vi "GenericIMAQSetConfig.vi"(8 "Show error dialog (F)":bool=TRUE, 10 "Camera":T1={"Framerate (Hz)"=100, "Exposure time (us)"=100, "Image size"={"Width"=1280, "Height"=1024}, "Number of buffers"=30}, 11 "IMAQ Session In":refnum<k11>) -> (3 "IMAQ Session Out":refnum<k11>)   [LabVIEW 2011]
uses:
  Main/Camera/GenericCameraConfigType.ctl
  Global_GenericIMAQCamera_HardwareConfig.vi
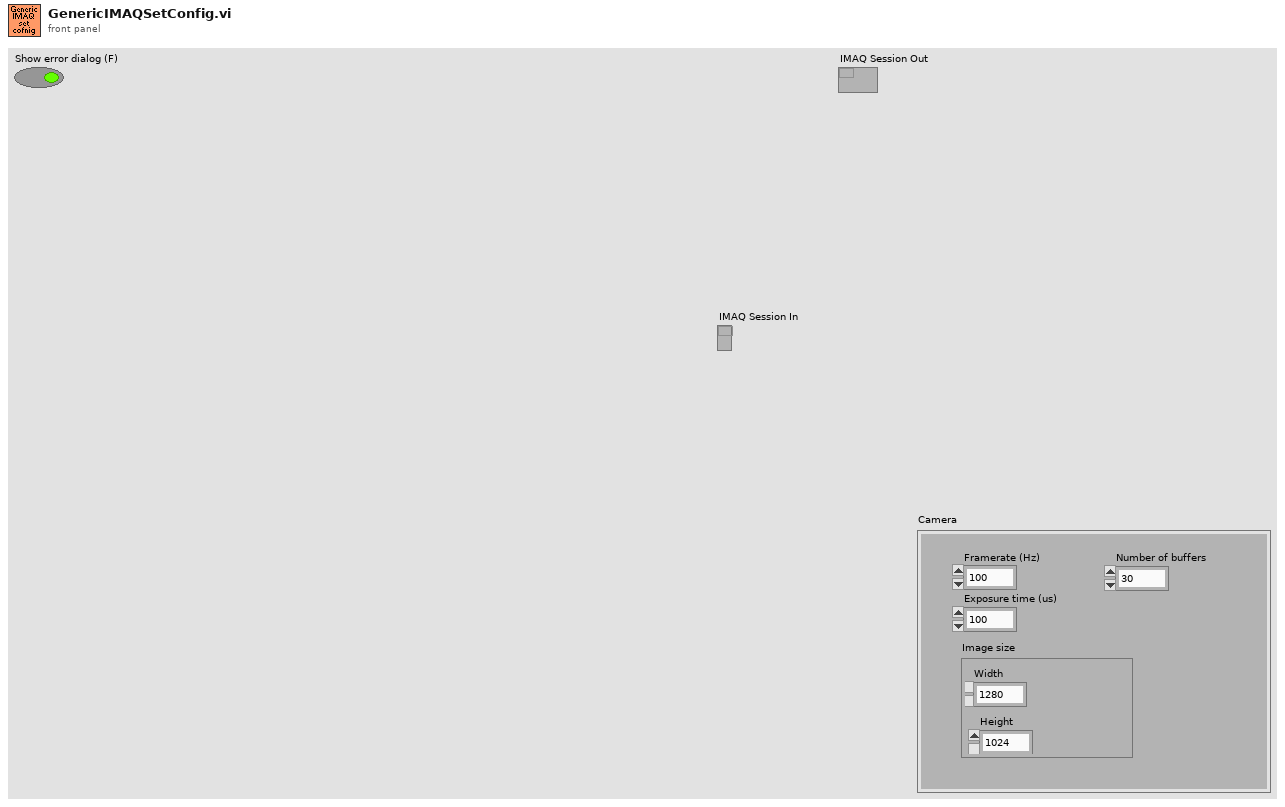
[diagram p1: front panel]
types:
  T1 = typedef "GenericCameraConfigType.ctl" = cluster{"Framerate (Hz)":i32, "Exposure time (us)":i32, "Image size":cluster{"Width":i32, "Height":i32}, "Number of buffers":i32}
  T2 = typedef "GenericIMAQHardwareConfig.ctl" = cluster{"Camera config mode":enum16{"Serial", "IMAQParam", "NoConfig"}, "Frame rate set cmd":string, "Exposure time set cmd":string, "Frame rate get cmd":string, "Exposure time get cmd":string, "IMAQ Identifier":string, "Serial return skip chars":i32, "Set width/height":string, "Set offset xy":string, "Get width":string, "Get height":string, "Get offset X":string, "Get offset Y":string, "Full frame size":cluster{"width":i32, "height":i32}}
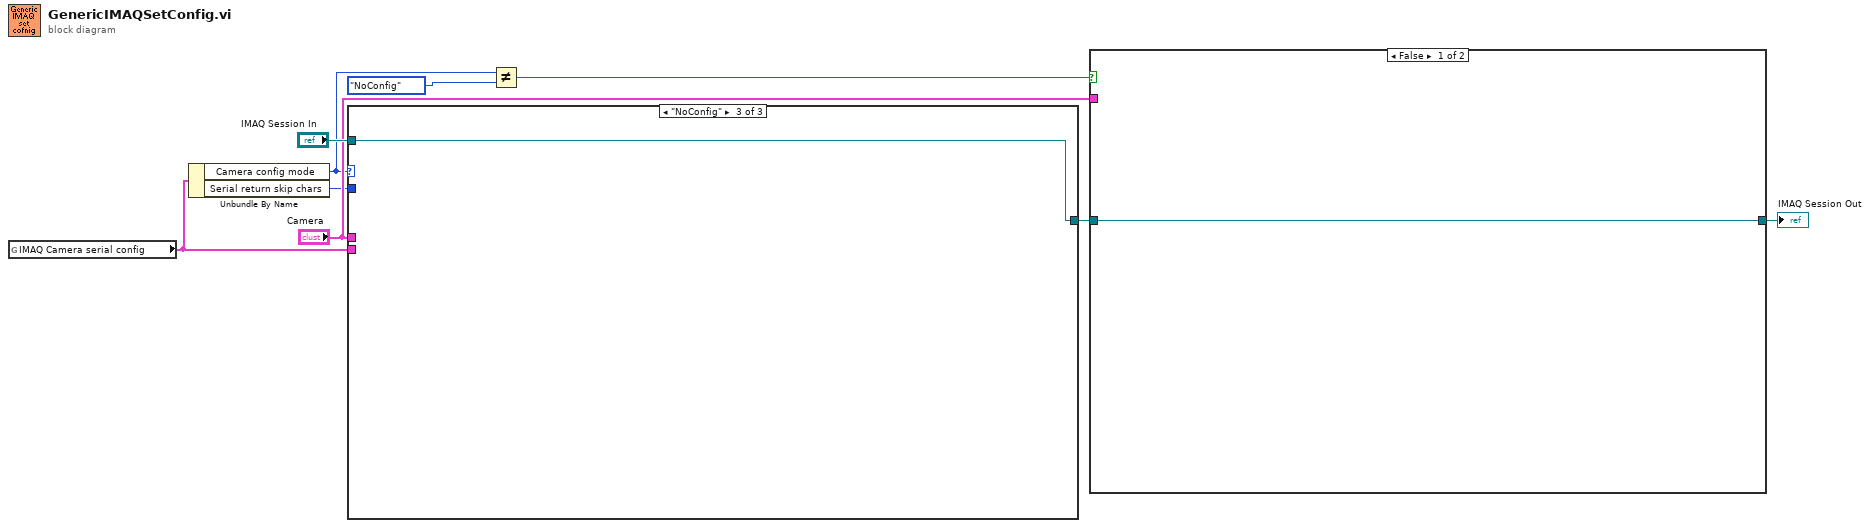
[diagram p0: block diagram]
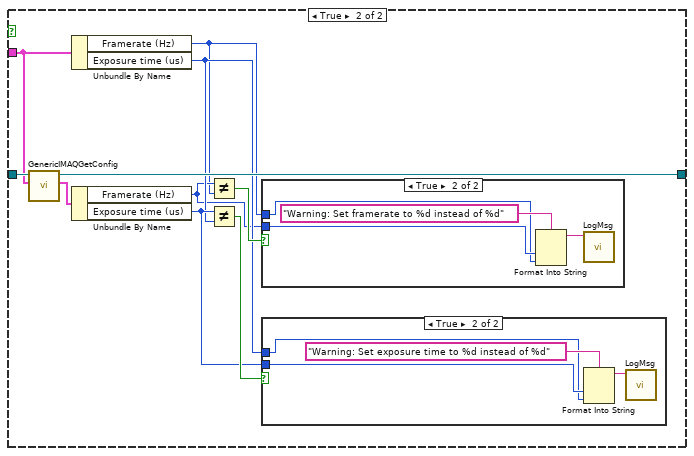
[diagram p2: hidden frame]
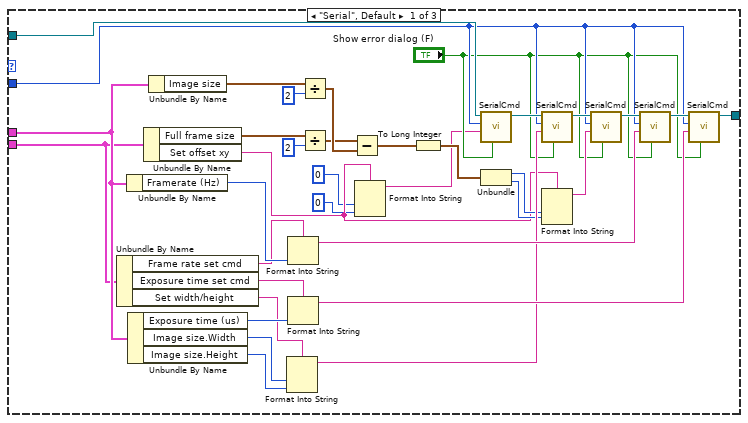
[diagram p5: hidden frame]
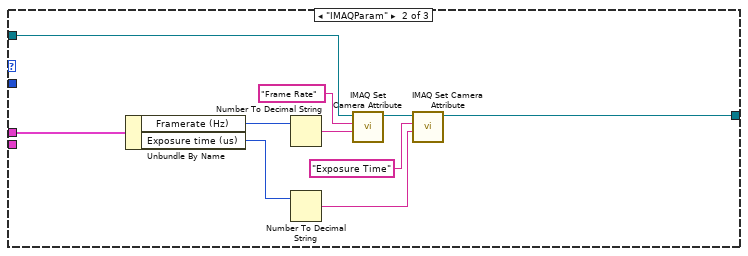
[diagram p6: hidden frame]
diagram:
  n1 = global read "Global_GenericIMAQCamera_HardwareConfig.vi" "IMAQ Camera serial config"() -> (w6:T2)
  n2 = Unbundle By Name(w6) -> ("Camera config mode"=w3:enum16{"Serial", "IMAQParam", "NoConfig"}, "Serial return skip chars"=w4:i32)
  n3 = case shown="\"NoConfig\"" w3 {
    tunnel: "IMAQ Session In" -> [w17 w54 w55]
    tunnel: [w44 w49 w55] -> w8
    tunnel: "Camera" -> [w22 w53 _]
    tunnel: w6 -> [w21 _ _]
    tunnel: w4 -> [w15 _ _]
    frame "Serial", Default {
      n4 = Unbundle By Name(w21) -> ("Frame rate set cmd"=w38:string, "Exposure time set cmd"=w37:string, "Set width/height"=w36:string)
      n5 = Unbundle By Name(w22) -> ("Framerate (Hz)"=w41:i32)
      n6 = Unbundle By Name(w22) -> ("Exposure time (us)"=w40:i32, "Image size.Width"=w35:i32, "Image size.Height"=w34:i32)
      n7 = Unbundle By Name(w21) -> ("Full frame size"=w23:cluster{"width":i32, "height":i32}, "Set offset xy"=w13:string)
      n8 = Unbundle By Name(w22) -> ("Image size"=w25:cluster{"Width":i32, "Height":i32})
      n9 = Format Into String(format string=w36, w35, w34) -> (resulting string=w33:string)  [unwired: 2 in, 1 out]
      n10 = Format Into String(format string=w38, w41) -> (resulting string=w42:string)  [unwired: 2 in, 1 out]
      n11 = Format Into String(format string=w37, w40) -> (resulting string=w39:string)  [unwired: 2 in, 1 out]
      n12 = Divide(x=w25, y=2) -> (x/y=w28:cluster{"Width":dbl, "Height":dbl})
      n13 = Divide(x=w23, y=2) -> (x/y=w27:cluster{"width":dbl, "height":dbl})
      n14 = Subtract(x=w27, y=w28) -> (x-y=w31:cluster{dbl, dbl})
      n15 = Format Into String(format string=w13, 0 ("input 1"), 0 ("input 2")) -> (resulting string=w10:string)  [unwired: 2 in, 1 out]
      n16 = To Long Integer(number=w31) -> (32bit integer=w32:cluster{i32, i32})
      n17 = call "SerialCmd.vi"("Show error dialog (T)"="Show error dialog (F)", "command"=w10, "Return string skip chars (2)"=w15, "IMAQ Refnum in"=w17) -> ("IMAQ Session Out"=w16:refnum<k11>)  [unwired: 4 in, 3 out]
      n18 = Unbundle(w32) -> (w29:i32, w30:i32)
      n19 = call "SerialCmd.vi"("Show error dialog (T)"="Show error dialog (F)", "command"=w33, "Return string skip chars (2)"=w15, "IMAQ Refnum in"=w16) -> ("IMAQ Session Out"=w20:refnum<k11>)  [unwired: 4 in, 3 out]
      n20 = Format Into String(format string=w13, w29, w30) -> (resulting string=w19:string)  [unwired: 2 in, 1 out]
      n21 = call "SerialCmd.vi"("Show error dialog (T)"="Show error dialog (F)", "command"=w19, "Return string skip chars (2)"=w15, "IMAQ Refnum in"=w20) -> ("IMAQ Session Out"=w18:refnum<k11>)  [unwired: 4 in, 3 out]
      n22 = call "SerialCmd.vi"("Show error dialog (T)"="Show error dialog (F)", "command"=w42, "Return string skip chars (2)"=w15, "IMAQ Refnum in"=w18) -> ("IMAQ Session Out"=w43:refnum<k11>)  [unwired: 4 in, 3 out]
      n23 = call "SerialCmd.vi"("Show error dialog (T)"="Show error dialog (F)", "command"=w39, "Return string skip chars (2)"=w15, "IMAQ Refnum in"=w43) -> ("IMAQ Session Out"=w44:refnum<k11>)  [unwired: 4 in, 3 out]
    }
    frame "IMAQParam" {
      n24 = Unbundle By Name(w53) -> ("Framerate (Hz)"=w52:i32, "Exposure time (us)"=w51:i32)
      n25 = Number To Decimal String(number=w52) -> (decimal integer string=w48:string)  [unwired: 1 in]
      n26 = Number To Decimal String(number=w51) -> (decimal integer string=w45:string)  [unwired: 1 in]
      n27 = call <vilib>:"IMAQ Set Camera Attribute.vi"("Attribute Value"=w48, "Camera Attribute"="Frame Rate", "IMAQ Session In"=w54) -> ("IMAQ Session Out"=w50:refnum<k11>)  [unwired: 5 in, 1 out]
      n28 = call <vilib>:"IMAQ Set Camera Attribute.vi"("Attribute Value"=w45, "Camera Attribute"="Exposure Time", "IMAQ Session In"=w50) -> ("IMAQ Session Out"=w49:refnum<k11>)  [unwired: 5 in, 1 out]
    }
    frame "NoConfig" {
    }
  }
  n29 = Not Equal?(x=w3, y=enum16{"Serial", "IMAQParam", "NoConfig"}."NoConfig") -> (x != y?=w1:bool)
  n30 = case shown="False" w1 {
    tunnel: w8 -> [w56 w66]
    tunnel: [w56 w65] -> w7
    tunnel: "Camera" -> [_ w57]
    frame False {
    }
    frame True {
      n31 = call "GenericIMAQGetConfig.vi"("Camera (in)"=w57, "IMAQ Refnum in"=w66) -> ("Camera"=w64:T1, "IMAQ Session Out"=w65:refnum<k11>)  [unwired: 8 in]
      n32 = Unbundle By Name(w57) -> ("Framerate (Hz)"=w58:i32, "Exposure time (us)"=w60:i32)
      n33 = Unbundle By Name(w64) -> ("Framerate (Hz)"=w59:i32, "Exposure time (us)"=w61:i32)
      n34 = Not Equal?(x=w59, y=w58) -> (x != y?=w63:bool)
      n35 = Not Equal?(x=w61, y=w60) -> (x != y?=w62:bool)
      n36 = case shown="True" w63 {
        tunnel: w59 -> [_ w72]
        tunnel: w58 -> [_ w71]
        frame False {
        }
        frame True {
          n37 = Format Into String(format string="Warning: Set framerate to %d instead of %d" ("msg"), w72, w71) -> (resulting string=w74:string)  [unwired: 2 in, 1 out]
          n38 = call "LogMsg.vi"("msg"=w74) -> ()  [unwired: 11 in]
        }
      }
      n39 = case shown="True" w62 {
        tunnel: w61 -> [_ w68]
        tunnel: w60 -> [_ w67]
        frame False {
        }
        frame True {
          n40 = Format Into String(format string="Warning: Set exposure time to %d instead of %d" ("msg"), w68, w67) -> (resulting string=w69:string)  [unwired: 2 in, 1 out]
          n41 = call "LogMsg.vi"("msg"=w69) -> ()  [unwired: 11 in]
        }
      }
    }
  }
  "IMAQ Session Out" <- w7
